vi "Tiepie-takeData-2018-06-01.vi"(0 "left rank":i32=2, 1 "right rank":i32=-1, 2 "deBaseline":bool, 3 "Thresh":dbl format="%#_13g", 4 "Laser parameter":T3, 5 "error in (no error)":errorcluster, 7 "ADC parameter":T1) -> (6 "output cluster":cluster{dbl[], "filtered data":dbl[]}, 8 "error out":errorcluster)   [LabVIEW 2013]
uses:
  cal_p.vi
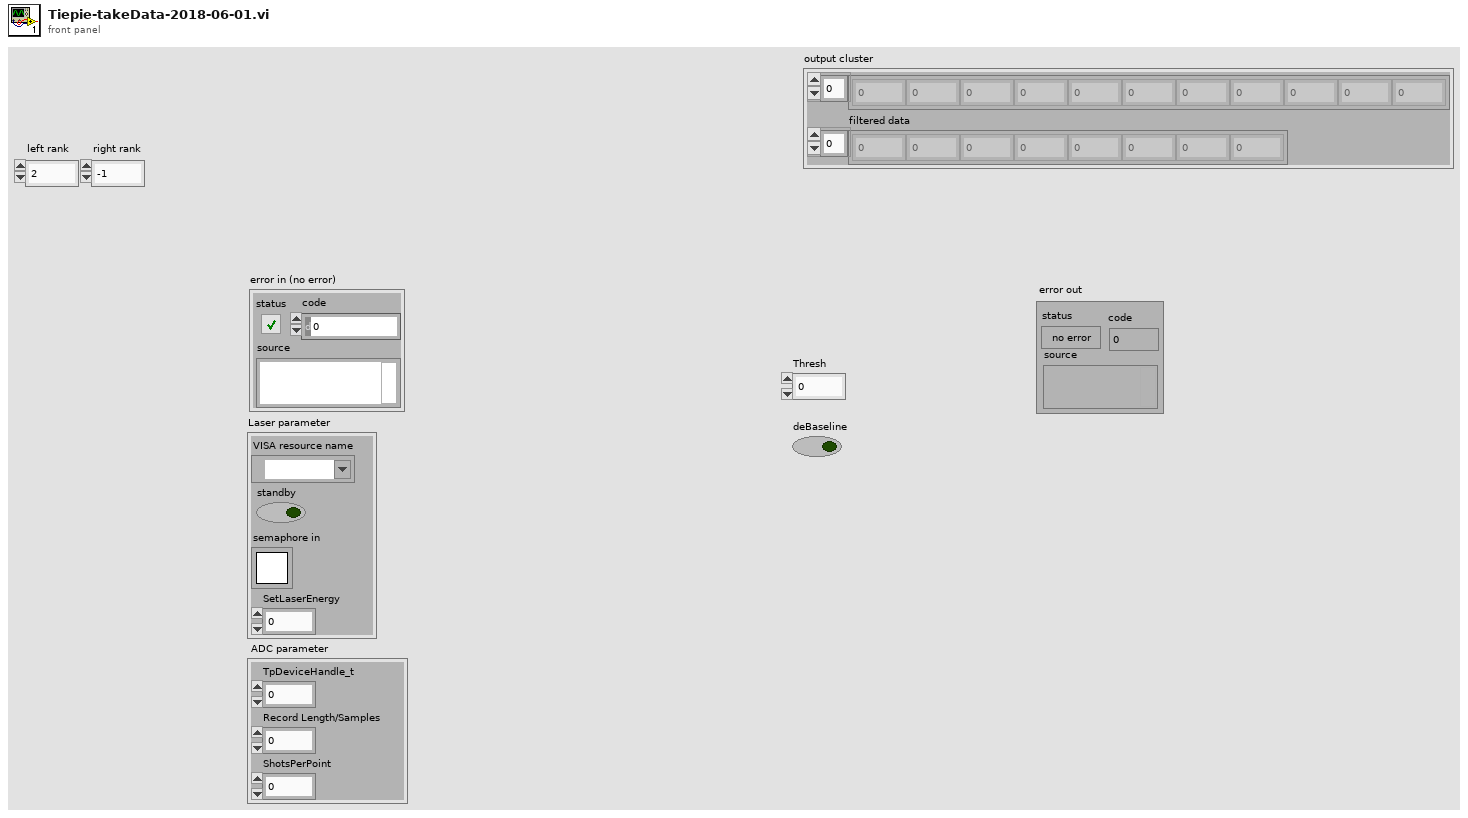
[diagram p1: front panel]
types:
  T1 = cluster{"TpDeviceHandle_t":u32, "Record Length/Samples":u64, "ShotsPerPoint":u16}
  T2 = typedef "Semaphore RefNum" = refnum<k1>
  T3 = cluster{"VISA resource name":refnum<visa-resource-name>, "standby":bool, "semaphore in":T2, "SetLaserEnergy":dbl}
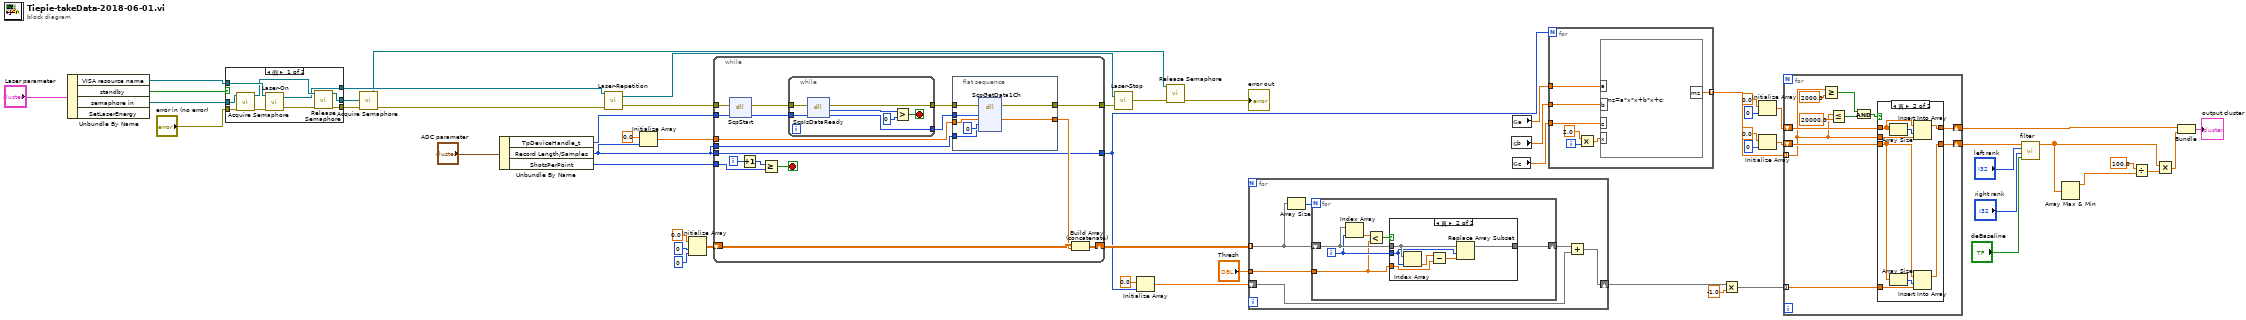
[diagram p0: block diagram]
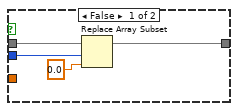
[diagram p3: hidden frame]
diagram:
  n1 = Unbundle By Name("Laser parameter") -> ("VISA resource name"=w43:refnum<visa-resource-name>, "standby"=w42:bool, "semaphore in"=w48:T2)  [unwired: 1 out]
  n2 = case shown="假" w42 {
    tunnel: "error in (no error)" -> [w63 w64]
    tunnel: w48 -> [w62 w65]
    tunnel: w43 -> [w59 w66]
    tunnel: [w57 w64] -> w40
    tunnel: [w56 w65] -> w41
    tunnel: [w55 w66] -> w39
    frame False {
      n3 = call <vilib>:"Acquire Semaphore.vi"("error in (no error)"=w63, "semaphore"=w62) -> ("error out"=w61:errorcluster, "semaphore out"=w58:T2)  [unwired: 3 in, 1 out]
      n4 = call "Laser-On.vi"("error in (no error)"=w61, "VISA resource name"=w59) -> ("error out"=w60:errorcluster, "VISA resource name out"=w55:refnum<visa-resource-name>)  [unwired: 2 in]
      n5 = call <vilib>:"Release Semaphore.vi"("error in (no error)"=w60, "semaphore"=w58) -> ("error out"=w57:errorcluster, "semaphore out"=w56:T2)  [unwired: 4 in]
    }
    frame True {
    }
  }
  n6 = call <vilib>:"Acquire Semaphore.vi"("error in (no error)"=w40, "semaphore"=w41) -> ("error out"=w38:errorcluster, "semaphore out"=w26:T2)  [unwired: 3 in, 1 out]
  n7 = Unbundle By Name("ADC parameter") -> ("TpDeviceHandle_t"=w46:u32, "Record Length/Samples"=w20:u64, "ShotsPerPoint"=w45:u16)
  n8 = call "Laser-Repetition.vi"("error in (no error)"=w38, "VISA resource name"=w39) -> ("error out"=w27:errorcluster, "VISA resource name out"=w37:refnum<visa-resource-name>)  [unwired: 2 in]
  n9 = Initialize Array(0.0, w20) -> (w51:dbl[])
  n10 = Initialize Array(0.0 ("element"), 0 ("dimension size"), 0 ("dimension size")) -> (w53:dbl[][])
  n11 = while {
    tunnel: w46 -> [w83]
    shift-right: [w68] -> w34
    shift-left: w53 -> [w70]
    tunnel: w20 -> [w75]
    tunnel: w51 -> [w74]
    tunnel: w45 -> [w73]
    tunnel: [w72] -> w28
    tunnel: w27 -> [w71]
    tunnel: w20 -> [w67]
    tunnel: [w67] -> w18
    i -> [w80]
    stop <- w76 stop-if-true
    n12 = dll-call lib="PTH1abs CUsers82158Desktop\nä¸æµ·é¡¹ç®2ä¸æµ·é¡¹ç®-2018-05-26ä¸æµ·é¡¹ç®-2018-05-26TOF software\tæ°æ®å¡\nlibtiepie.dll" fn="ScpStart"(error in=w71, "TpDeviceHandle_t"=w83) -> (error out=w82:errorcluster, "TpDeviceHandle_t"=w81:u32)  [unwired: 3 in, 1 out]
    n13 = Increment(x=w80) -> (x+1=w79:i32)
    n14 = Greater Or Equal?(x=w79, y=w73) -> (x >= y?=w76:bool)
    n15 = while {
      tunnel: w82 -> [w97]
      tunnel: w81 -> [w96]
      tunnel: [w95] -> w78
      tunnel: [w94] -> w77
      stop <- w91 stop-if-true
      n16 = dll-call lib="PTH1abs CUsers82158Desktop\nä¸æµ·é¡¹ç®2ä¸æµ·é¡¹ç®-2018-05-26ä¸æµ·é¡¹ç®-2018-05-26TOF software\tæ°æ®å¡\nlibtiepie.dll" fn="ScpIsDataReady"(error in=w97, "TpDeviceHandle_t"=w96) -> (error out=w95:errorcluster, "DataReady"=w92:u8, "TpDeviceHandle_t"=w94:u32)  [unwired: 2 in, 1 out]
      n17 = Greater?(x=w92, y=0 ("index")) -> (0:w91:bool)
    }
    n18 = flat-sequence {
      tunnel: [w90] -> w69
      tunnel: w78 -> [w89]
      tunnel: w77 -> [w88]
      tunnel: w75 -> [w86]
      tunnel: w74 -> [w85]
      tunnel: [w84] -> w72
      frame #0 {
        n19 = dll-call lib="PTH1abs CUsers82158Desktop\nä¸æµ·é¡¹ç®2ä¸æµ·é¡¹ç®-2018-05-26ä¸æµ·é¡¹ç®-2018-05-26TOF software\tæ°æ®å¡\nlibtiepie.dll" fn="ScpGetData1Ch"(error in=w89, "TpDeviceHandle_t"=w88, "pBufferCh1"=w85, "qwStartIndex"=u64 0, "qwSampleCount"=w86) -> (error out=w84:errorcluster, "pBufferCh1"=w90:sgl[])  [unwired: 6 in, 1 out]
      }
    }
    n20 = Build Array (concatenate)(w70, w69) -> (w68:dbl[][])
  }
  n21 = call "Laser-Stop.vi"("error in (no error)"=w28, "VISA resource name"=w37) -> ("error out"=w44:errorcluster)
  n22 = Initialize Array(0.0 ("element"), w18) -> (w32:dbl[])
  n23 = call <vilib>:"Release Semaphore.vi"("error in (no error)"=w44, "semaphore"=w26) -> ("error out"=→"error out":errorcluster)  [unwired: 4 in, 1 out]
  n24 = for {
    tunnel: w34 -> [w103] mode=indexing
    shift-right: [w101] -> w30
    shift-left: w32 -> [w100]
    tunnel: "Thresh" -> [w98]
    n25 = Array Size(array=w103) -> (size(s)=w102:i32)
    n26 = for {
      N: w102 -> [_]
      shift-right: [w107] -> w99
      shift-left: w103 -> [w106]
      tunnel: w98 -> [w104]
      i -> [w105]
      n27 = Index Array(array=w106, index=w105) -> (element=w109:dbl)
      n28 = Less?(x=w109, y=w104) -> (x < y?=w108:bool)
      n29 = case shown="真" w108 {
        tunnel: [w111 w114] -> w107
        tunnel: w106 -> [w113 w119]
        tunnel: w105 -> [w112 w115]
        tunnel: w104 -> [_ w117]
        frame False {
          n30 = Replace Array Subset "Replace Array Subset"(array=w113, new element=0.0 ("new element/subarray"), index=w112) -> (w111:dbl[])
        }
        frame True {
          n31 = Index Array(array=w119, index=w115) -> (element=w118:dbl)
          n32 = Subtract(x=w118, y=w117) -> (x-y=w116:dbl)
          n33 = Replace Array Subset(array=w119, new element=w116, index=w115) -> (w114:dbl[])
        }
      }
    }
    n34 = Add(x=w99, y=w100) -> (x+y=w101:dbl[])
  }
  n35 = global read "cal_p.vi" "b"() -> (w22:dbl)
  n36 = global read "cal_p.vi" "a"() -> (w23:dbl)
  n37 = global read "cal_p.vi" "c"() -> (w21:dbl)
  n38 = for {
    N: w18 -> [_]
    tunnel: [w126] -> w16 mode=indexing
    tunnel: w21 -> [w123]
    tunnel: w22 -> [w124]
    tunnel: w23 -> [w125]
    i -> [w122]
    n39 = Multiply(x=2.0, y=w122) -> (x*y=w120:dbl)
    n40 = formula code="mz=a*x*x+b*x+c;"("a"=w125, "b"=w124, "c"=w123, "x"=w120) -> ("mz"=w126:dbl)
  }
  n41 = Multiply(x=w30, y=-1.0) -> (x*y=w8:dbl[])
  n42 = Initialize Array(0.0 ("element"), 0 ("dimension size")) -> (w11:dbl[])
  n43 = Initialize Array(0.0 ("element"), 0 ("dimension size")) -> (w10:dbl[])
  n44 = for {
    tunnel: w16 -> [w129] mode=indexing
    tunnel: w8 -> [w130] mode=indexing
    shift-right: [w127] -> w6
    shift-left: w10 -> [w131]
    shift-right: [w128] -> w9
    shift-left: w11 -> [w132]
    n45 = Greater Or Equal?(x=w129, y=2000.0) -> (x >= y?=w135:bool)
    n46 = Less Or Equal?(x=w129, y=20000.0) -> (x <= y?=w136:bool)
    n47 = And(x=w135, y=w136) -> (x .and. y?=w133:bool)
    n48 = case shown="真" w133 {
      tunnel: w132 -> [w139 w147]
      tunnel: w131 -> [w138 w146]
      tunnel: w130 -> [_ w143]
      tunnel: w129 -> [_ w142]
      tunnel: [w138 w141] -> w127
      tunnel: [w139 w140] -> w128
      frame False {
      }
      frame True {
        n49 = Array Size(array=w147) -> (size(s)=w144:i32)
        n50 = Array Size(array=w146) -> (size(s)=w145:i32)
        n51 = Insert Into Array(array=w147, index=w144, new element=w142) -> (w140:dbl[])
        n52 = Insert Into Array(array=w146, index=w145, new element=w143) -> (w141:dbl[])
      }
    }
  }
  n53 = call "filter.vi"("deBaseline"="deBaseline", "right rank"="right rank", "left rank"="left rank", "data"=w6) -> ("filtered data"=w2:dbl[])  [unwired: 7 in]
  n54 = Array Max & Min(array=w2) -> (max value=w4:dbl)  [unwired: 3 out]
  n55 = Divide(x=100.0, y=w4) -> (x/y=w3:dbl)
  n56 = Multiply(x=w2, y=w3) -> (x*y=w1:dbl[])
  n57 = Bundle(w9, w1) -> (→"output cluster":cluster{dbl[], dbl[]})  [unwired: 1 in]
